vi "Max Button Process.vi"(8 "error in (no error)":errorcluster, 11 "UI_Top_Customer in":refnum<class "UI_Top_Customer.lvclass">) -> (0 "error out":errorcluster, 3 "UI_Top_Customer out":refnum<class "UI_Top_Customer.lvclass">)   [LabVIEW 2021, in "UI_Top_Customer.lvclass"]
uses:
  UI_Top_Customer.lvclass
  C:/Program Files (x86)/National Instruments/LabVIEW 2021/user.lib/John_Lib/AbstractActorTemplate/AbstractActorTemplate/UIActorTop.lvclass
  <userlib>/John_Lib/Control/Panel State.ctl
  UI_Top_Customer.lvclass/UI_Top_Customer.ctl
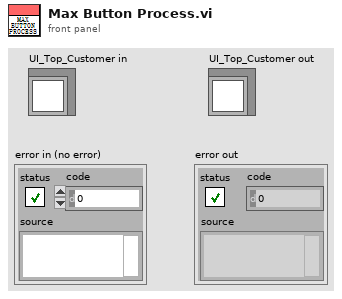
[diagram p1: front panel]
types:
  T1 = typedef "Panel State.ctl" = string
  T2 = enum32{"Invalid", "Standard", "Closed", "Hidden", "Minimized", "Maximized"}
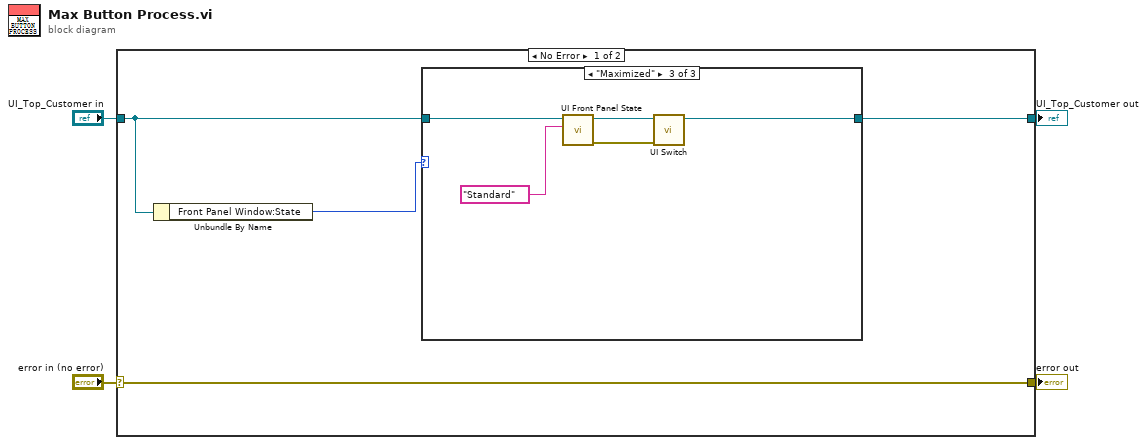
[diagram p0: block diagram]
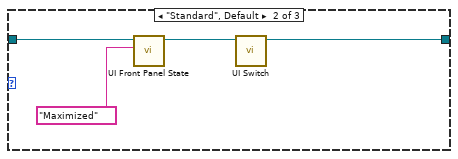
[diagram p3: hidden frame]
diagram:
  n1 = case shown="No Error" "error in (no error)" {
    selector: "error in (no error)" -> [w8 w20]
    tunnel: [w8 w20] -> w3
    tunnel: [w7 w19] -> w1
    tunnel: "UI_Top_Customer in" -> [w5 w19]
    frame No Error {
      n2 = Unbundle By Name(w5) -> ("Front Panel Window:State"=w6:T2)
      n3 = case shown="\"Maximized\"" w6 {
        tunnel: w5 -> [w9 w13 w18]
        tunnel: [w9 w10 w15] -> w7
        frame "Invalid" {
        }
        frame "Standard", Default {
          n4 = call-dynamic "UI Front Panel State.vi"("Argument"=T1 "Maximized", "UI ActorTop in"=w13) -> ("UI ActorTop out"=w11:refnum<class "UI_Top_Customer.lvclass">)  [unwired: 8 in, 1 out]
          n5 = call "UI Switch.vi"("UI_Top_Customer in"=w11) -> ("UI_Top_Customer out"=w10:refnum<class "UI_Top_Customer.lvclass">)  [unwired: 9 in, 1 out]
        }
        frame "Maximized" {
          n6 = call-dynamic "UI Front Panel State.vi"("Argument"=T1 "Standard", "UI ActorTop in"=w18) -> ("error out"=w14:errorcluster, "UI ActorTop out"=w16:refnum<class "UI_Top_Customer.lvclass">)  [unwired: 8 in]
          n7 = call "UI Switch.vi"("error in (no error)"=w14, "UI_Top_Customer in"=w16) -> ("UI_Top_Customer out"=w15:refnum<class "UI_Top_Customer.lvclass">)  [unwired: 8 in, 1 out]
        }
      }
    }
    frame Error {
    }
  }
  "error out" <- w3
  "UI_Top_Customer out" <- w1
